vi "gmail71.vi"() -> ()   [LabVIEW 2010]
panel:
  out "error out":errorcluster
  in  "CC (Carbon Copy Recipient - Optional)":string
  in  "Attachment - Optional":path
  in  "Port":i32=2525
  in  "Enable SSL":bool
  in  "GMAIL Account Password":string="antonebut"
  in  "GMAIL Account User ID (eg: jsmity77)":string="decent"
  in  "Outgoing Mail Server (SMTP)":string="smtp.ngs.ru"
  in  "Body":string="It works!"
  in  "Subject":string="Sending test Email"
  in  "Recipient's Name":string="Anton"
  in  "Recipient's Email Address Address":string="tone@ngs.ru"
  in  "Sender's Name":string="Tone"
  in  "Sender's Email Address (eg: jsmith77@gmail.com)":string="decent@ngs.ru"
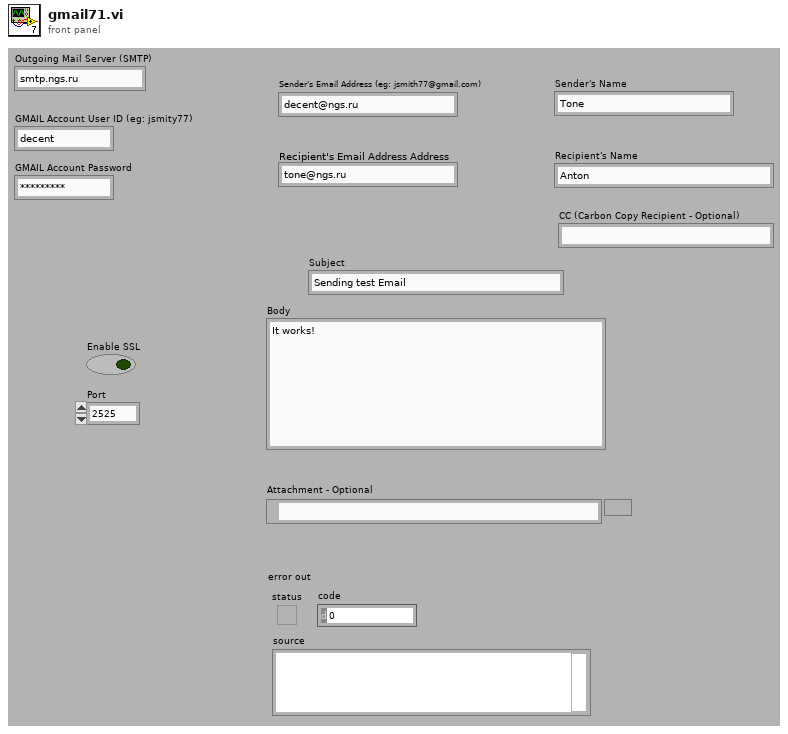
[diagram p1: front panel]
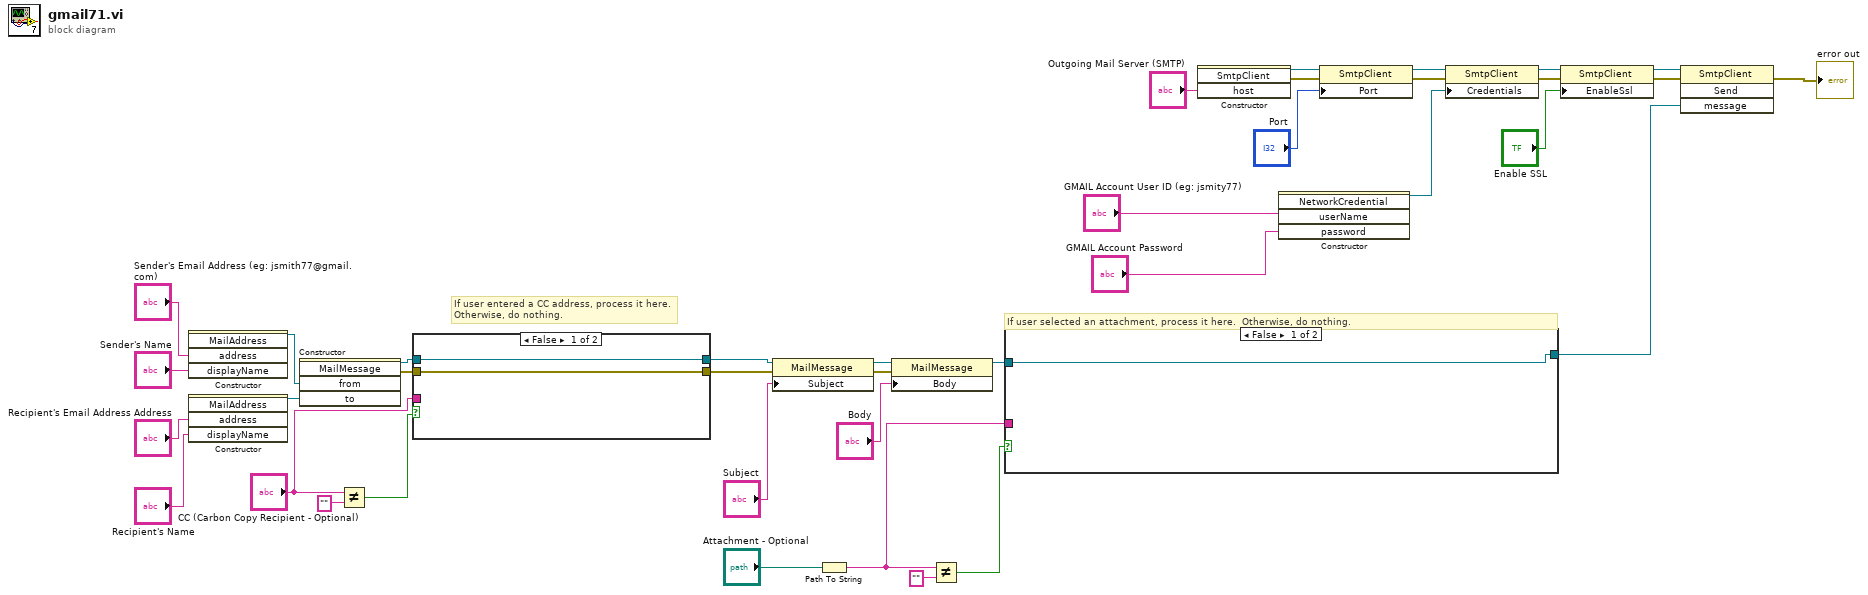
[diagram p0: block diagram]
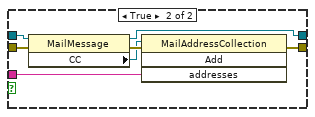
[diagram p2: hidden frame]
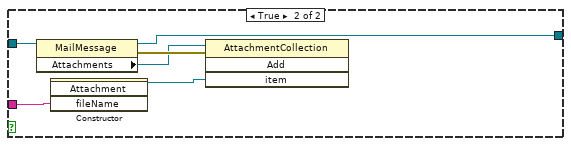
[diagram p3: hidden frame]
diagram:
  # "If user selected an attachment, process it here.  Otherwise, do nothing."
  # "If user entered a CC address, process it here.\nOtherwise, do nothing."
  n1 = constructor class="MailAddress"("address"="Sender's Email Address (eg: jsmith77@gmail.com)", "displayName"="Sender's Name") -> (reference out=w37:refnum<k24>)  [unwired: 3 in, 4 out]
  n2 = constructor class="MailAddress"("address"="Recipient's Email Address Address", "displayName"="Recipient's Name") -> (reference out=w38:refnum<k24>)  [unwired: 3 in, 4 out]
  n3 = constructor class="MailMessage"("from"=w37, "to"=w38) -> (reference out=w5:refnum<k24>, error out=w4:errorcluster)  [unwired: 3 in, 3 out]
  n4 = Not Equal?(x="CC (Carbon Copy Recipient - Optional)", y="") -> (x != y?=w7:bool)
  n5 = case shown="False" w7 {
    tunnel: "CC (Carbon Copy Recipient - Optional)" -> [_ w45]
    tunnel: w5 -> [w40 w44]
    tunnel: w4 -> [w39 w43]
    tunnel: [w40 w42] -> w3
    tunnel: [w39 w41] -> w2
    frame False {
    }
    frame True {
      n6 = property class="MailMessage"(reference=w44, error in=w43) -> (reference out=w42:refnum<k24>, error out=w47:errorcluster, "CC"=w46:refnum<k24>)
      n7 = invoke class="MailAddressCollection" method="Add"(reference=w46, error in=w47, "addresses"=w45) -> (error out=w41:errorcluster)  [unwired: 1 in, 3 out]
    }
  }
  n8 = property class="MailMessage"(reference=w3, error in=w2, "Subject"="Subject") -> (reference out=w28:refnum<k24>, error out=w36:errorcluster)
  n9 = Path To String(path="Attachment - Optional") -> (string=w9:string)
  n10 = property class="MailMessage"(reference=w28, error in=w36, "Body"="Body") -> (reference out=w14:refnum<k24>)  [unwired: 1 out]
  n11 = Not Equal?(x=w9, y="") -> (x != y?=w10:bool)
  n12 = case shown="False" w10 {
    tunnel: w14 -> [w48 w51]
    tunnel: [w48 w50] -> w13
    tunnel: w9 -> [_ w49]
    frame False {
    }
    frame True {
      n13 = property class="MailMessage"(reference=w51) -> (reference out=w50:refnum<k24>, error out=w54:errorcluster, "Attachments"=w52:refnum<k24>)  [unwired: 1 in]
      n14 = constructor class="Attachment"("fileName"=w49) -> (reference out=w53:refnum<k24>)  [unwired: 3 in, 3 out]
      n15 = invoke class="AttachmentCollection" method="Add"(reference=w52, error in=w54, "item"=w53) -> ()  [unwired: 1 in, 4 out]
    }
  }
  n16 = constructor class="SmtpClient"("host"="Outgoing Mail Server (SMTP)") -> (reference out=w22:refnum<k24>, error out=w18:errorcluster)  [unwired: 3 in, 2 out]
  n17 = constructor class="NetworkCredential"("userName"="GMAIL Account User ID (eg: jsmity77)", "password"="GMAIL Account Password") -> (reference out=w23:refnum<k24>)  [unwired: 3 in, 4 out]
  n18 = property class="SmtpClient"(reference=w22, error in=w18, "Port"="Port") -> (reference out=w21:refnum<k24>, error out=w17:errorcluster)
  n19 = property class="SmtpClient"(reference=w21, error in=w17, "Credentials"=w23) -> (reference out=w20:refnum<k24>, error out=w16:errorcluster)
  n20 = property class="SmtpClient"(reference=w20, error in=w16, "EnableSsl"="Enable SSL") -> (reference out=w19:refnum<k24>, error out=w15:errorcluster)
  n21 = invoke class="SmtpClient" method="Send"(reference=w19, error in=w15, "message"=w13) -> (error out=→"error out":errorcluster)  [unwired: 1 in, 3 out]
